vi "Ocatve Based Sub-Bands (32k).vi"(1 "Array":dbl[](array[numeric])) -> (0 "Sub-Band's":T1)   [LabVIEW 2013]
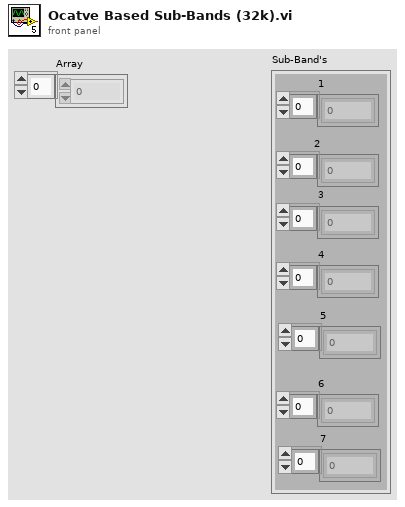
[diagram p1: front panel]
types:
  T1 = cluster{"1":dbl[], "2":dbl[], "3":dbl[], "4":dbl[], "5":dbl[], "6":dbl[], "7":dbl[]}
  T2 = cluster{dbl[], dbl[], dbl[], dbl[], dbl[], dbl[], dbl[]}
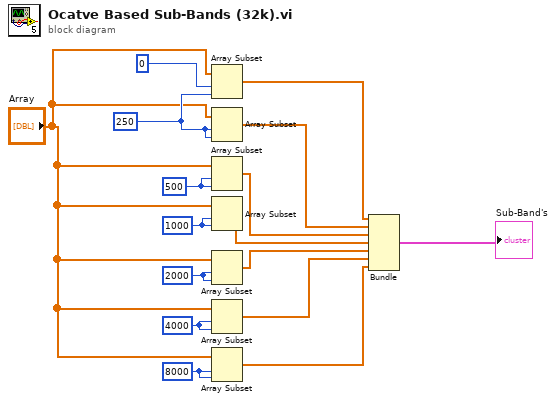
[diagram p0: block diagram]
diagram:
  w10 = 8000 ("length")
  w11 = 4000 ("length")
  w12 = 2000 ("length")
  w13 = 1000 ("length")
  w14 = 500 ("length")
  w15 = 250 ("length")
  n1 = Array Subset(array="Array", index=0, length=w15) -> (w9:dbl[])
  n2 = Array Subset(array="Array", index=w15, length=w15) -> (w8:dbl[])
  n3 = Array Subset(array="Array", index=w14, length=w14) -> (w6:dbl[])
  n4 = Array Subset(array="Array", index=w13, length=w13) -> (w5:dbl[])
  n5 = Array Subset(array="Array", index=w12, length=w12) -> (w4:dbl[])
  n6 = Array Subset(array="Array", index=w11, length=w11) -> (w3:dbl[])
  n7 = Array Subset(array="Array", index=w10, length=w10) -> (w2:dbl[])
  n8 = Bundle(w9, w8, w6, w5, w4, w3, w2) -> (→"Sub-Band's":T2)  [unwired: 1 in]
